vi "Analyzer.Timer.vi"(8 "error in (no error)":errorcluster, 10 "Queue":refnum<queue>, 11 "Analyzer in":refnum<class "Analyzer.lvclass">) -> (0 "error out":errorcluster)   [LabVIEW 2022 SP3, in "Analyzer.lvclass"]
uses:
  Analyzer.lvclass
  Typedefs/PublicEvents--Analyzer.NewEventMessage.ctl
  Analyzer.lvclass/Analyzer.ctl
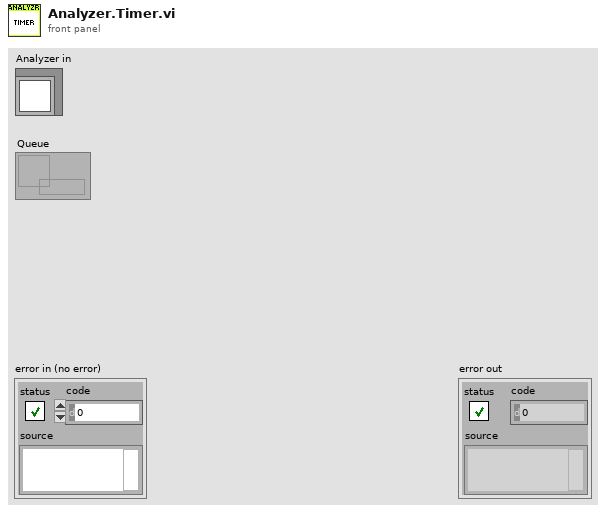
[diagram p1: front panel]
types:
  T1 = typedef "Analyzer.lvclass/PublicEvents--Analyzer.NewEventMessage.ctl" = cluster{"Title":string, "Message":variant}
  T2 = cluster{"Reset":bool, "Elapsed Time (s)":dbl, "State":string, "Self Ref":refnum<class "Analyzer.lvclass">}
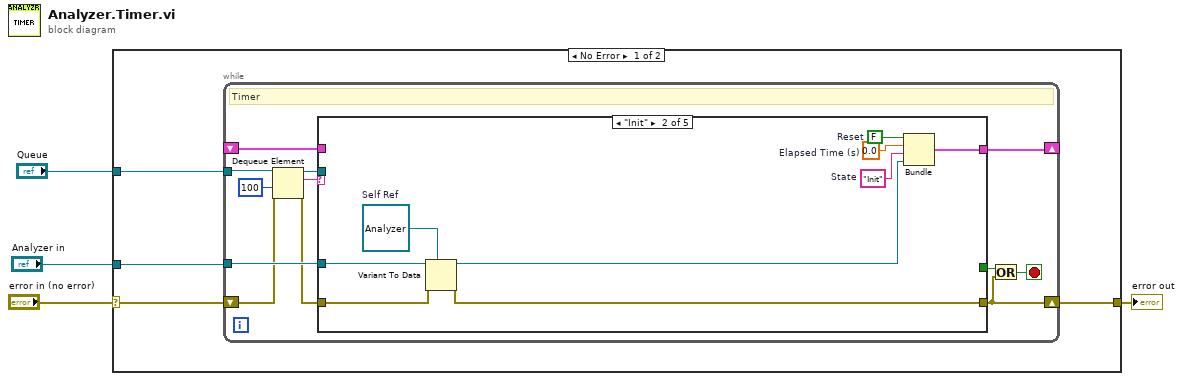
[diagram p0: block diagram]
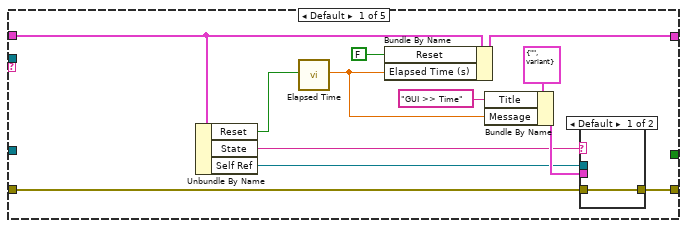
[diagram p2: hidden frame]
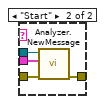
[diagram p3: hidden frame]
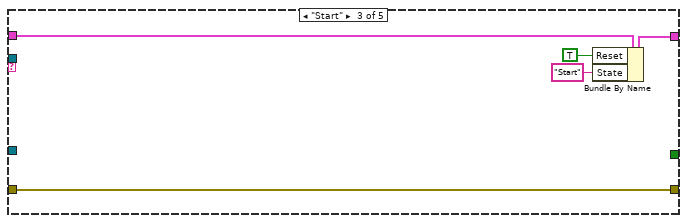
[diagram p4: hidden frame]
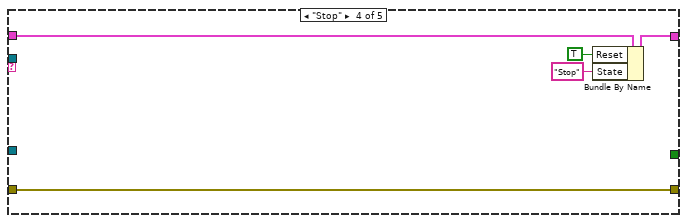
[diagram p5: hidden frame]
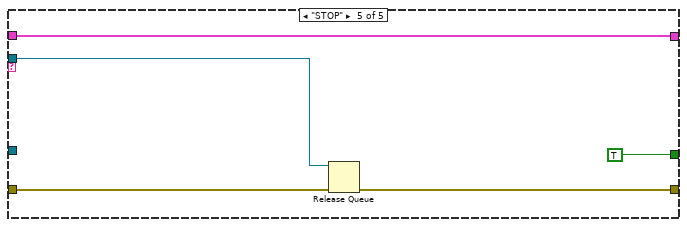
[diagram p6: hidden frame]
diagram:
  n1 = case shown="No Error" "error in (no error)" {
    selector: "error in (no error)" -> [w7 w62]
    tunnel: [w6 w62] -> w3
    tunnel: "Analyzer in" -> [w5 _]
    tunnel: "Queue" -> [w8 _]
    frame No Error {
      n2 = while {
        tunnel: w8 -> [w20]
        shift-right: [w18] -> _
        shift-left: _ -> [w17]
        tunnel: w5 -> [w15]
        shift-right: [w12] -> w6
        shift-left: w7 -> [w11]
        stop <- w14 stop-if-true
        # "Timer"
        n3 = Dequeue Element(queue=w20, timeout in ms (-1)=100, error in (no error)=w11) -> (queue out=w9:refnum<queue>, element=w19:string, error out=w10:errorcluster)  [unwired: 1 out]
        n4 = case shown="\"Init\"" w19 {
          tunnel: [_ _ _ _ TRUE] -> w13
          tunnel: [w31 w46 w50 w55 w60] -> w18
          tunnel: w17 -> [w32 _ w51 w56 w60]
          tunnel: w15 -> [_ w42 _ _ _]
          tunnel: [w25 w40 w48 w53 w58] -> w12
          tunnel: w10 -> [w24 w41 w48 w53 w59]
          tunnel: w9 -> [_ _ _ _ w57]
          frame Default {
            n5 = Unbundle By Name(w32) -> ("Reset"=w21:bool, "State"=w22:string, "Self Ref"=w23:refnum<class "Analyzer.lvclass">)
            n6 = call "Elapsed Time"("Reset"=w21) -> ("Elapsed Time (s)"=w27:dbl)  [unwired: 11 in, 7 out]
            n7 = Bundle By Name(cluster=w32, "Reset"=FALSE, "Elapsed Time (s)"=w27) -> (w31:T2)
            n8 = Bundle By Name(cluster=T1 {"Title"="", "Message"=variant} ("event data"), "Title"="GUI >> Time", "Message"=w27) -> (w26:T1)
            n9 = case shown="Default" w22 {
              tunnel: w26 -> [_ w37]
              tunnel: [w33 w36] -> w25
              tunnel: w24 -> [w33 w35]
              tunnel: w23 -> [_ w34]
              frame Default {
              }
              frame "Start" {
                n10 = call "Analyzer.NewMessage.vi"("error in (no error)"=w35, "event data"=w37, "Analyzer in"=w34) -> ("error out"=w36:errorcluster)  [unwired: 7 in, 1 out]
              }
            }
          }
          frame "Init" {
            w38 = "Init"  # State
            w43 = refnum<class "Analyzer.lvclass"> refnum  # Self Ref
            w45 = FALSE  # Reset
            w44 = 0.0  # Elapsed Time (s)
            n11 = Variant To Data(error in=w41, type=w43, Variant=w42) -> (data=w39:refnum<class "Analyzer.lvclass">, error out=w40:errorcluster)
            n12 = Bundle("Reset"=w45, "Elapsed Time (s)"=w44, "State"=w38, "Self Ref"=w39) -> (w46:T2)  [unwired: 1 in]
          }
          frame "Start" {
            n13 = Bundle By Name(cluster=w51, "Reset"=TRUE ("Start"), "State"="Start") -> (w50:T2)
          }
          frame "Stop" {
            n14 = Bundle By Name(cluster=w56, "Reset"=TRUE ("Start"), "State"="Stop") -> (w55:T2)
          }
          frame "STOP" {
            n15 = Release Queue(queue=w57, error in (no error)=w59) -> (error out=w58:errorcluster)  [unwired: 1 in, 2 out]
          }
        }
        n16 = Or(x=w13, y=w12) -> (x .or. y?=w14:bool)
      }
    }
    frame Error {
    }
  }
  "error out" <- w3
